vi "GE 5565PIORC.Registers.INTCSR.Local DMA Channel 0 Interrupt Enable.Get.vi"(8 "error in (no error)":errorcluster, 11 "GE 5565PIORC in":refnum<class "GE 5565PIORC.lvclass">) -> (0 "error out":errorcluster, 2 "Local DMA Channel 0 Interrupt Enable":bool, 3 "GE 5565PIORC out":refnum<class "GE 5565PIORC.lvclass">)   [LabVIEW 2020, in "GE 5565PIORC.lvclass"]
doc: "Writing a one (1) enables DMA Channel 0 interrupts. Clearing the DMA status bit also clears the interrupt."
uses:
  GE 5565PIORC.lvclass
  GE 5565PIORC.Registers.Local Configuration.ctl
  GE 5565PIORC.lvclass/GE 5565PIORC.ctl
  GE 5565PIORC.Registers.Local Configuration.Read (U32).vi
  Methods/GE 5565PIORC.Bit Manipulation.Get Bit (U32).vi
  Methods/GE 5565PIORC.Registers.Read.vi
  Methods/GE 5565PIORC.Registers.Read (U32).vi
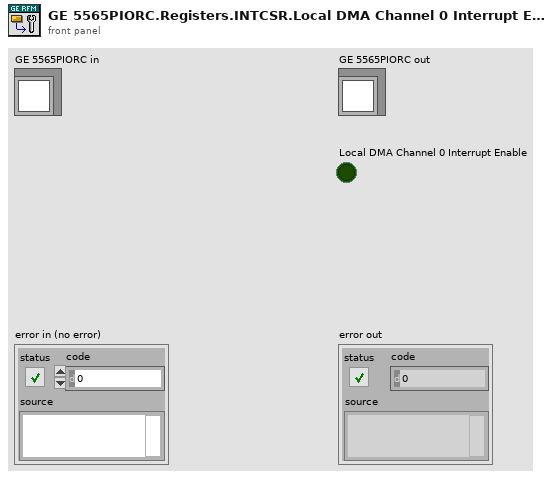
[diagram p1: front panel]
types:
  T1 = typedef "GE 5565PIORC.lvclass/GE 5565PIORC.Registers.Local Configuration.ctl" = u32
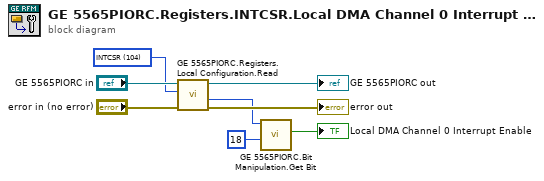
[diagram p0: block diagram]
diagram:
  w4 = T1 104 items=["MARBR"=8, "BIGEND"=12, "INTCSR"=104, "PCIHREV"=116, "DMAMODE0"=128, "DMAPADR0"=132, "DMALADR0"=136, "DMASIZ0"=140, "DMADPR0"=144, "DMACSR0"=168, "DMADAC0"=180, "LAS1RR"=240, "LAS1BA"=244] ("Local Configuration Registers")
  n1 = call-poly "GE 5565PIORC.Registers.Local Configuration.Read.vi"("error in (no error)"="error in (no error)", "Register"=w4, "GE 5565PIORC in"="GE 5565PIORC in") -> ("error out"=→"error out":errorcluster, "Value"=w3:u32, "GE 5565PIORC out"=→"GE 5565PIORC out":refnum<class "GE 5565PIORC.lvclass">)  [unwired: 6 in]
  n2 = call-poly "GE 5565PIORC.Bit Manipulation.Get Bit.vi"("bit index"=18, "packed value in"=w3) -> ("bit"=→"Local DMA Channel 0 Interrupt Enable":bool)  [unwired: 8 in, 1 out]
